vi "Filter Event Data.vi"(8 "error in (no error)":errorcluster, 10 "EventFilter Reference":T1, 11 "ControlDragSourceUpdateMsg In":refnum<class "ControlDragSourceUpdateMsg.lvclass">) -> (0 "error out":errorcluster, 2 "Discard?":bool, 3 "ControlDragSourceUpdateMsg Out":refnum<class "ControlDragSourceUpdateMsg.lvclass">)   [LabVIEW 2018, in "MVA Framework.lvlib" / "ActorEvents.lvlib" / "ControlDragSourceUpdateMsg.lvclass"]
uses:
  ControlDragSourceUpdateMsg.lvclass
  IEventFilter/IEventFilter.lvclass
  IEventFilter/EventFilter Reference.ctl
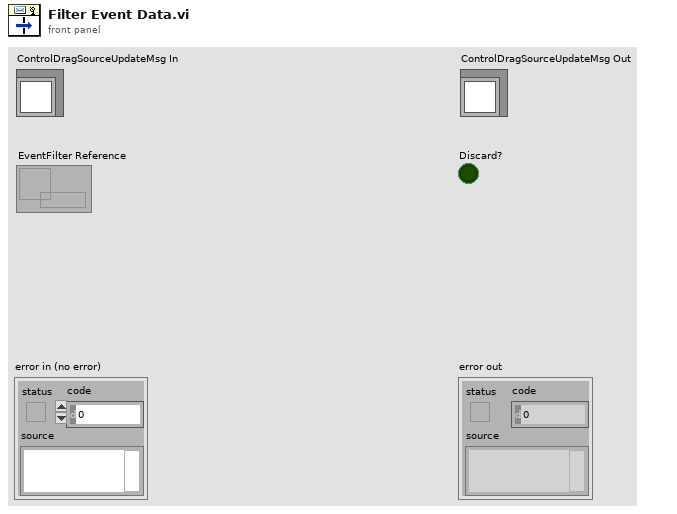
[diagram p1: front panel]
types:
  T1 = typedef "MVA Framework.lvlib/ActorEvents.lvlib/IEventFilter.lvclass/EventFilter Reference.ctl" = refnum<data-value>
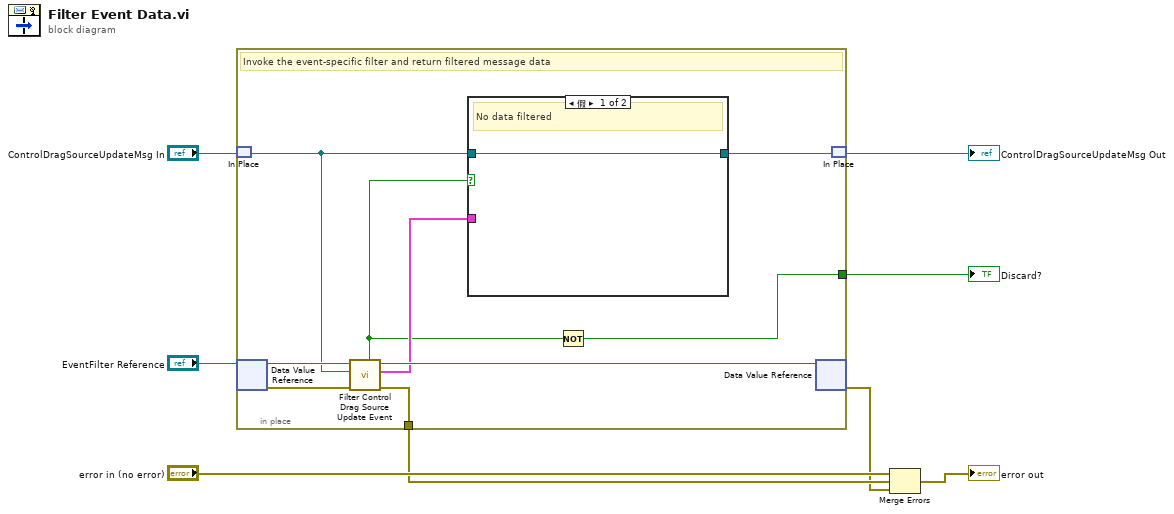
[diagram p0: block diagram]
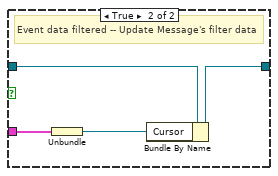
[diagram p2: hidden frame]
diagram:
  n1 = in-place {
    in-place-border: [w14] -> w5
    in-place-border: [w9] -> w3
    # "Invoke the event-specific filter and return filtered message data"
    n2 = in-place-match #1("ControlDragSourceUpdateMsg In") -> (w12:refnum<class "ControlDragSourceUpdateMsg.lvclass">)
    n3 = in-place-dvr #2("EventFilter Reference") -> (w17:refnum<class "IEventFilter.lvclass">, w15:errorcluster)
    n4 = call-dynamic "Filter Control Drag Source Update Event.vi"("error in (no error)"=w15, "ControlDragSourceUpdateMsg"=w12, "IEventFilter in"=w17) -> ("error out"=w14:errorcluster, "Filtered Event Data"=w13:cluster{"Cursor":refnum<k1>}, "IEventFilter out"=w16:refnum<class "IEventFilter.lvclass">, "Data Filtered?"=w10:bool)  [unwired: 4 in, 1 out]
    n5 = case shown="假" w10 {
      tunnel: w13 -> [_ w20]
      tunnel: w12 -> [w18 w22]
      tunnel: [w18 w21] -> w11
      frame False {
        # "No data filtered"
      }
      frame True {
        # "Event data filtered -- Update Message's filter data"
        n6 = Unbundle(w20) -> ("Cursor"=w19:refnum<k1>)
        n7 = Bundle By Name(cluster=w22, "Cursor"=w19) -> (w21:refnum<class "ControlDragSourceUpdateMsg.lvclass">)
      }
    }
    n8 = Not(x=w10) -> (.not. x?=w9:bool)
    n9 = in-place-dvr #2(w16) -> (w4:errorcluster)  [unwired: 1 out]
    n10 = in-place-match #1(w11) -> (→"ControlDragSourceUpdateMsg Out":refnum<class "ControlDragSourceUpdateMsg.lvclass">)
  }
  "Discard?" <- w3
  n11 = Merge Errors("error in (no error)", w5, w4) -> (→"error out":errorcluster)
